vi "KE6221 -- Set Wave External Trig Params.vi"(0 "Resource In":refnum<visa-resource-name>, 1 "Check For SCPI Errors? (T)":bool=TRUE, 7 "External Trig Params In":T1={"Ext Trig Enabled?"=FALSE, "Trig Link In Line"=enum."None", "Inactive Level (%)"=50.0, "Ignore Retrigs?"=FALSE} {"Inactive Level (%)" min=-100.0 max=100.0 format="%.3p"}, 11 "error in (no error)":errorcluster, 12 "Read Back Set Values? (T)":bool=TRUE) -> (4 "Resource Out (dupl)":refnum<visa-resource-name>, 8 "External Trig Params Out":T1={"Ext Trig Enabled?"=FALSE, "Trig Link In Line"=enum."None", "Inactive Level (%)"=50.0, "Ignore Retrigs?"=FALSE} {"Inactive Level (%)" min=-100.0 max=100.0 format="%.3p"}, 15 "error out":errorcluster)   [LabVIEW 2019, in "Keithley 622x.lvlib"]
doc: "Sets the trigger parameters for waveform playback. Note that this VI can only be used with the 6221, since the 6220 doesn't support this feature."
uses:
  Keithley 622x.lvlib
  Typedefs/KE6221 -- Wave External Trig Params.ctl
  Low Level/Typedefs/KE6221 -- Wave Extern Trig Link In Line.ctl
  Low Level/Typedefs/KE6221 -- Wave Inactive Level.ctl
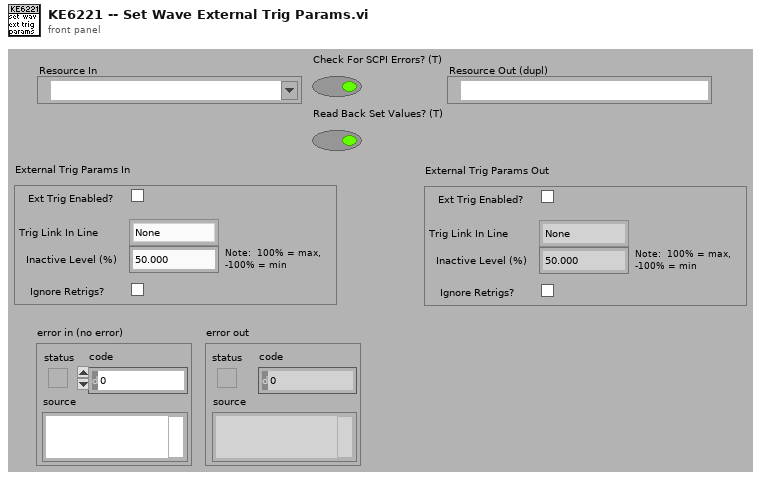
[diagram p1: front panel]
types:
  T1 = typedef "Keithley 622x.lvlib/KE6221 -- Wave External Trig Params.ctl" = cluster{"Ext Trig Enabled?":bool, "Trig Link In Line":T2, "Inactive Level (%)":T3, "Ignore Retrigs?":bool}
  T2 = typedef "Keithley 622x.lvlib/KE6221 -- Wave Extern Trig Link In Line.ctl" = enum16{"None", "1", "2", "3", "4", "5", "6"}
  T3 = typedef "Keithley 622x.lvlib/KE6221 -- Wave Inactive Level.ctl" = dbl
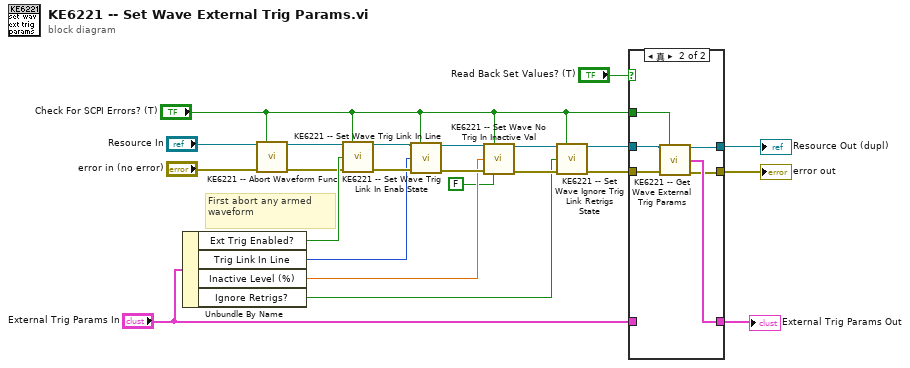
[diagram p0: block diagram]
diagram:
  # "First abort any armed\nwaveform"
  n1 = Unbundle By Name("External Trig Params In") -> ("Ext Trig Enabled?"=w14:bool, "Trig Link In Line"=w13:T2, "Inactive Level (%)"=w12:T3, "Ignore Retrigs?"=w11:bool)
  n2 = call "KE6221 -- Abort Waveform Func.vi"("Resource In"="Resource In", "Check For SCPI Errors? (T)"="Check For SCPI Errors? (T)", "error in (no error)"="error in (no error)") -> ("Resource Out (dupl)"=w2:refnum<visa-resource-name>, "error out"=w3:errorcluster)  [unwired: 11 in]
  n3 = call "KE6221 -- Set Wave Trig Link In Enab State.vi"("Resource In"=w2, "Check For SCPI Errors? (T)"="Check For SCPI Errors? (T)", "Trig Link In Enabled?"=w14, "error in (no error)"=w3) -> ("Resource Out (dupl)"=w23:refnum<visa-resource-name>, "error out"=w22:errorcluster)  [unwired: 10 in]
  n4 = call "KE6221 -- Set Wave Trig Link In Line.vi"("Resource In"=w23, "Check For SCPI Errors? (T)"="Check For SCPI Errors? (T)", "Trig Link In Line"=w13, "error in (no error)"=w22) -> ("Resource Out (dupl)"=w21:refnum<visa-resource-name>, "error out"=w20:errorcluster)  [unwired: 10 in]
  n5 = call "KE6221 -- Set Wave No Trig In Inactive Val.vi"("Resource In"=w21, "Check For SCPI Errors? (T)"="Check For SCPI Errors? (T)", "Inactive Level In (%)"=w12, "error in (no error)"=w20, "Read Back Set Value? (T)"=FALSE) -> ("Resource Out (dupl)"=w19:refnum<visa-resource-name>, "error out"=w18:errorcluster)  [unwired: 8 in, 1 out]
  n6 = call "KE6221 -- Set Wave Ignore Trig Link Retrigs State.vi"("Resource In"=w19, "Check For SCPI Errors? (T)"="Check For SCPI Errors? (T)", "Ignore Retrigs?"=w11, "error in (no error)"=w18) -> ("Resource Out (dupl)"=w16:refnum<visa-resource-name>, "error out"=w15:errorcluster)  [unwired: 10 in]
  n7 = case shown="真" "Read Back Set Values? (T)" {
    tunnel: w16 -> [w25 w32]
    tunnel: w15 -> [w24 w31]
    tunnel: "Check For SCPI Errors? (T)" -> [_ w30]
    tunnel: "External Trig Params In" -> [w26 _]
    tunnel: [w26 w29] -> w8
    tunnel: [w25 w27] -> w7
    tunnel: [w24 w28] -> w6
    frame False {
    }
    frame True {
      n8 = call "KE6221 -- Get Wave External Trig Params.vi"("Resource In"=w32, "Check For SCPI Errors? (T)"=w30, "error in (no error)"=w31) -> ("Resource Out (dupl)"=w27:refnum<visa-resource-name>, "External Trig Params"=w29:T1, "error out"=w28:errorcluster)  [unwired: 10 in]
    }
  }
  "Resource Out (dupl)" <- w7
  "error out" <- w6
  "External Trig Params Out" <- w8
